vi "add data indicies controls.vi"(8 "error in":errorcluster, 9 "Channels to create":T1[](array[typedef]), 10 "runtime class path":path, 11 "Application in":refnum<vi>) -> (0 "error out":errorcluster, 2 "cfg class base path out":path)   [LabVIEW 2013, in "FixedChannelTBModuleDecideFeatures.lvclass"]
uses:
  FixedChannelTBModuleDecideFeatures.lvclass
  channel configuration.ctl
  <vilib>/NI/Tag Bus Module Framework/channel/channel classification.ctl
  <vilib>/NI/Tag Bus/tag/Data Type.ctl
  <vilib>/NI/Tag Bus Module Framework/channel/TBM channel.lvclass
  <vilib>/NI/Tag Bus/tag/tag descriptor.lvclass
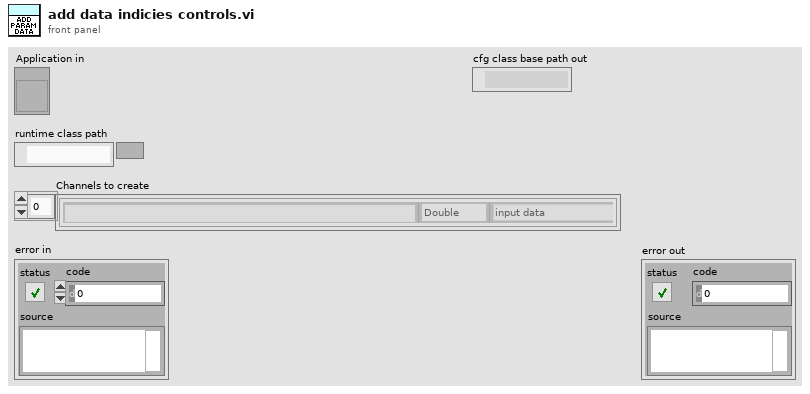
[diagram p1: front panel]
types:
  T1 = typedef "FixedChannelTBModuleDecideFeatures.lvclass/channel configuration.ctl" = cluster{"Name":string, "channel classification":T2, "data type":T3}
  T2 = typedef "TBM channel.lvclass/channel classification.ctl" = enum16{"input data", "output data", "processing parameter", "processing result"}
  T3 = typedef "tag bus.lvlib/tag descriptor.lvclass/Data Type.ctl" = enum16{"Double", "Single", "I64", "I32", "I16", "I8", "U64", "U32", "U16", "U8", "Boolean", "String", "Array of Double", "Array of Single", "Array of I64", "Array of I32", "Array of I16", "Array of I8", "Array of U64", "Array of U32", "Array of U16", "Array of U8", "Array of Boolean", "Array of String"}
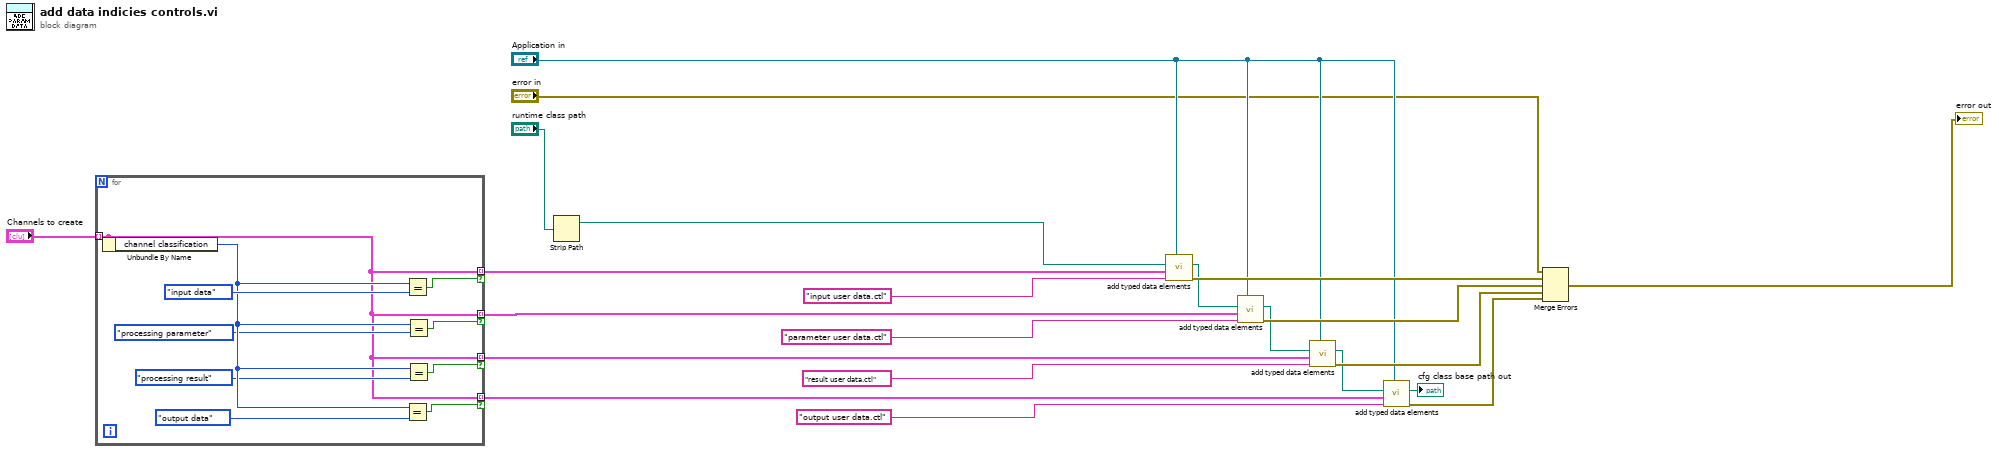
[diagram p0: block diagram]
diagram:
  n1 = for {
    tunnel: "Channels to create" -> [w23] mode=indexing
    tunnel: [w23] -> w19 mode=indexing if=w31
    tunnel: [w23] -> w17 mode=indexing if=w30
    tunnel: [w23] -> w15 mode=indexing if=w28
    tunnel: [w23] -> w12 mode=indexing if=w29
    n2 = Unbundle By Name(w23) -> ("channel classification"=w27:T2)
    n3 = Equal?(x=w27, y=channel_classification."output data" ("x")) -> (x = y?=w29:bool)
    n4 = Equal?(x=w27, y=channel_classification."input data" ("x")) -> (x = y?=w31:bool)
    n5 = Equal?(x=w27, y=channel_classification."processing parameter" ("x")) -> (x = y?=w30:bool)
    n6 = Equal?(x=w27, y=channel_classification."processing result" ("x")) -> (x = y?=w28:bool)
  }
  n7 = Strip Path(path="runtime class path") -> (stripped path=w13:path)  [unwired: 1 out]
  n8 = call "add typed data elements.vi"("Application in"="Application in", "Typedef relative path"="input user data.ctl" ("name or relative path"), "Channels to create"=w19, "cfg class base path"=w13) -> ("error out"=w10:errorcluster, "cfg class base path out"=w4:path)  [unwired: 6 in]
  n9 = call "add typed data elements.vi"("Application in"="Application in", "Typedef relative path"="parameter user data.ctl" ("name or relative path"), "Channels to create"=w17, "cfg class base path"=w4) -> ("error out"=w9:errorcluster, "cfg class base path out"=w3:path)  [unwired: 6 in]
  n10 = call "add typed data elements.vi"("Application in"="Application in", "Typedef relative path"="result user data.ctl" ("name or relative path"), "Channels to create"=w15, "cfg class base path"=w3) -> ("error out"=w8:errorcluster, "cfg class base path out"=w2:path)  [unwired: 6 in]
  n11 = call "add typed data elements.vi"("Application in"="Application in", "Typedef relative path"="output user data.ctl" ("name or relative path"), "Channels to create"=w12, "cfg class base path"=w2) -> ("error out"=w7:errorcluster, "cfg class base path out"=→"cfg class base path out":path)  [unwired: 6 in]
  n12 = Merge Errors("error in", w10, w9, w8, w7) -> (→"error out":errorcluster)
